vi "Send.vi"(5 "Record Topic Name?":bool, 7 "Message Priority":T1, 8 "error in (no error)":errorcluster, 9 "Timeout":i32, 10 "Message":refnum<class "Message Interface.lvclass">, 11 "Message Transport Binding in":refnum<class "Message Transport Binding.lvclass">=refnum) -> (0 "error out":errorcluster, 2 "Timed Out?":bool, 3 "Message Transport Binding out":refnum<class "Message Transport Binding.lvclass">)   [LabVIEW 2016, in "Stream Mediator.lvlib" / "Message Transport Binding.lvclass"]
doc: "--\nCopyright © 2017 Composed SystemsI All rights reserved.\n\nAuthor: Jon McBee <jon.mcbee@composed.io>\n\nThis library is provided \"AS IS\" ,WITHOUT WARRANTIES OR\nCONDITIONS OF ANY KIND, either express or implied.\n\nComposed Systems -- composed.io\n\nStream 0.0.1.1\nJon McBee - Composed Systems\nCopyright (c) 2017, Composed Systems"
uses:
  <userlib>/Composed Systems/Stream/Mediator/Classes/Message Transport Binding/Message Transport Binding.lvclass
  C:/Program Files (x86)/National Instruments/LabVIEW 2016/user.lib/Composed Systems/Stream/Mediator/Classes/Message Transport Interface/Message Transport Interface.lvclass
  <userlib>/Composed Systems/Stream/Mediator/Classes/Message Interface/Message Interface.lvclass
  <userlib>/Composed Systems/Stream/Mediator/Classes/Message Transport Interface/Message Priority.ctl
  <userlib>/Composed Systems/Stream/Mediator/Classes/Message Interface/Message Interface.lvclass/Message Interface.ctl
  <userlib>/Composed Systems/Stream/Mediator/Classes/Message Transport Binding/Message Transport Binding.lvclass/Message Transport Binding.ctl
  <userlib>/Composed Systems/Stream/Mediator/Classes/Message Transport Interface/Message Transport Interface.lvclass
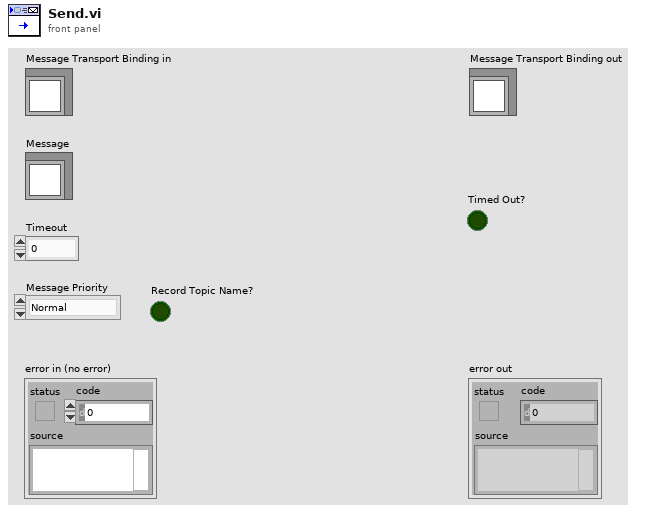
[diagram p1: front panel]
types:
  T1 = typedef "Stream Mediator.lvlib/Message Transport Interface.lvclass/Message Priority.ctl" = enum16{"Normal", "High"}
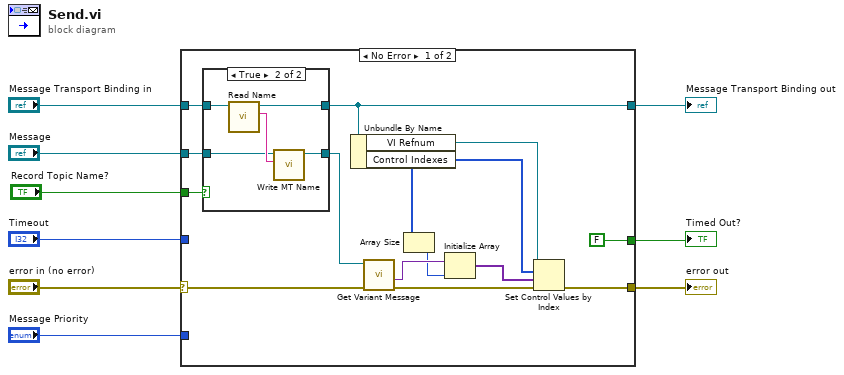
[diagram p0: block diagram]
diagram:
  n1 = case shown="No Error" "error in (no error)" {
    selector: "error in (no error)" -> [w22 w32]
    tunnel: "Message" -> [w12 _]
    tunnel: [w23 w32] -> w7
    tunnel: [w13 w31] -> w6
    tunnel: "Message Transport Binding in" -> [w14 w31]
    tunnel: "Message Priority" -> [_ _]
    tunnel: "Timeout" -> [_ _]
    tunnel: [FALSE _] -> w2
    tunnel: "Record Topic Name?" -> [w10 _]
    frame No Error {
      n2 = case shown="True" w10 {
        tunnel: w14 -> [w25 w29]
        tunnel: [w25 w28] -> w13
        tunnel: w12 -> [w24 w27]
        tunnel: [w24 w26] -> w11
        frame False {
        }
        frame True {
          n3 = call <userlib>:"Read Name.vi"("Message Transport Interface in"=w29) -> ("Name"=w30:string, "Message Transport Interface out"=w28:refnum<class "Message Transport Binding.lvclass">)  [unwired: 8 in, 1 out]
          n4 = call <userlib>:"Write MT Name.vi"("MT Name"=w30, "Message Interface in"=w27) -> ("Message Interface out"=w26:refnum<class "Message Interface.lvclass">)  [unwired: 9 in]
        }
      }
      n5 = Unbundle By Name(w13) -> ("VI Refnum"=w20:refnum<vi>, "Control Indexes"=w19:i32[])
      n6 = call-dynamic "Get Variant Message.vi"("error in (no error)"=w22, "Message Interface in"=w11) -> ("error out"=w21:errorcluster, "Value"=w18:variant)  [unwired: 6 in, 2 out]
      n7 = Array Size(array=w19) -> (size(s)=w17:i32)
      n8 = Initialize Array(w18, w17) -> (w16:variant[])
      n9 = Set Control Values by Index(0:w20, 1:w19, 2:w16, 3:w21) -> (11:w23:errorcluster)
    }
    frame Error {
    }
  }
  "error out" <- w7
  "Message Transport Binding out" <- w6
  "Timed Out?" <- w2
